vi "AMZ_S3_APIHLP_Multipart Upload Data to PartList XML.vi"(8 "error in (no error)":errorcluster, 11 "Multipart Upload Data":T1 {"Parts"."PartNumber" min=1 max=10000}) -> (0 "error out":errorcluster, 3 "PartList XML":string)   [LabVIEW 2015, in "LV Interface for Amazon S3.lvlib"]
uses:
  LV Interface for Amazon S3.lvlib
  Typedefs/AMZ_S3_Multipart Upload Data.ctl
  Typedefs/AMZ_S3_Multipart Upload Part Data.ctl
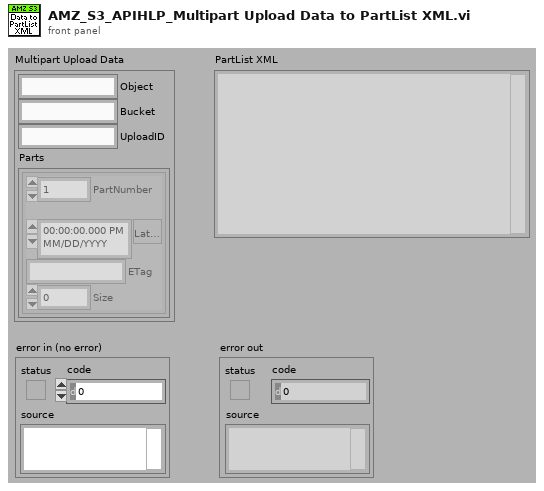
[diagram p1: front panel]
types:
  T1 = typedef "LV Interface for Amazon S3.lvlib/AMZ_S3_Multipart Upload Data.ctl" = cluster{"Object":string, "Bucket":string, "UploadID":string, "Parts":T2[]}
  T2 = typedef "LV Interface for Amazon S3.lvlib/AMZ_S3_Multipart Upload Part Data.ctl" = cluster{"PartNumber":u16, "Lat modified":timestamp, "ETag":string, "Size":u64}
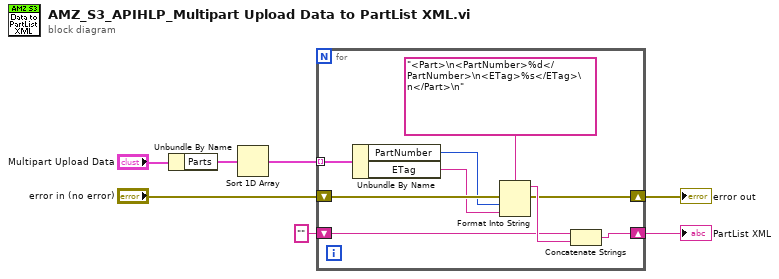
[diagram p0: block diagram]
diagram:
  n1 = Unbundle By Name("Multipart Upload Data") -> ("Parts"=w2:T2[])
  n2 = Sort 1D Array(array=w2) -> (sorted array=w1:T2[])
  n3 = for {
    tunnel: w1 -> [w16] mode=indexing
    shift-right: [w8] -> w4
    shift-left: "error in (no error)" -> [w14]
    shift-right: [w9] -> w3
    shift-left: "" -> [w10]
    n4 = Unbundle By Name(w16) -> ("PartNumber"=w13:u16, "ETag"=w12:string)
    n5 = Format Into String(format string="<Part>\n<PartNumber>%d</PartNumber>\n<ETag>%s</ETag>\n</Part>\n", error in=w14, w13, w12) -> (resulting string=w11:string, error out=w8:errorcluster)  [unwired: 1 in]
    n6 = Concatenate Strings(w10, w11) -> (w9:string)
  }
  "error out" <- w4
  "PartList XML" <- w3
